vi "Functional Imaging-16bit display mapping.vi"(8 "error in (no error)":errorcluster) -> (0 "error out":errorcluster)   [LabVIEW 2013]
uses:
  Global variables/gl_Functional Imaging-Global variables.vi
panel:
  out "16-bit Display Mapping:All Elements":T1
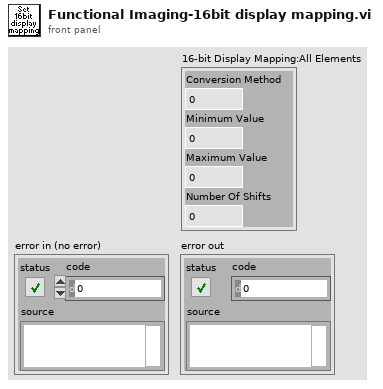
[diagram p1: front panel]
types:
  T1 = cluster{"Conversion Method":u32, "Minimum Value":i32, "Maximum Value":i32, "Number Of Shifts":i32}
  T2 = typedef "Functional Imging UI Refs.ctl" = cluster{"Menu ref":refnum<k9>, "Image control":refnum<vi>, "VI ref":refnum<vi>, "XGrapher":refnum<vi>, "Smoothing":refnum<vi>, "POI Averaging":refnum<vi>, "Normalize":refnum<vi>, "POI data points in each trial":refnum<vi>, "Channel":refnum<vi>, "Experiment data folder path":refnum<vi>, "[ROI vis]":refnum<vi>, "[Groups] visbl":T3, "Group Name":refnum<vi>, "POI index":refnum<vi>, "Trial No.":refnum<vi>, "Intensity Zoom":refnum<vi>, "Trial Cursor Enabled":refnum<vi>, "Number of Trials (ind 1)":refnum<vi>, "Number of Trials (ind 2)":refnum<vi>, "MiniScans Available":refnum<vi>, "POI Available":refnum<vi>, "Defer graph updates":refnum<vi>, "Waveform selector":refnum<vi>, "#of selected POI":refnum<vi>, "#of selected MiniScans":refnum<vi>, "#of selected groups":refnum<vi>, "Max Z-Projection":refnum<vi>, "Z-Plane Selector":refnum<vi>, "Index of miniscan point to visualise":refnum<vi>, "ROI vis. mode":refnum<vi>, "Total # of points":refnum<vi>, "Index of group clicked on":refnum<vi>, "Pane 1":refnum<vi>, "Pane 2":refnum<vi>, "Pane 3":refnum<vi>, "Pane 4":refnum<vi>, "Pane 5":refnum<vi>, "Pane 6":refnum<vi>, "Deselect all ROI":refnum<vi>, "Deselect all groups":refnum<vi>}
  T3 = typedef "Groups array referecne.ctl" = refnum<vi>
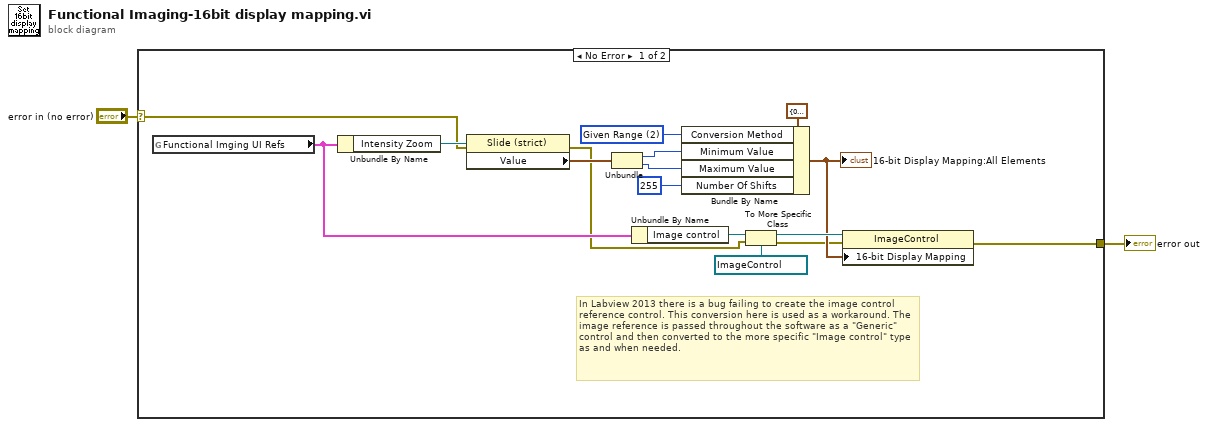
[diagram p0: block diagram]
diagram:
  n1 = case shown="No Error" "error in (no error)" {
    selector: "error in (no error)" -> [w3 w19]
    tunnel: [w4 w19] -> w2
    frame No Error {
      w16 = u32 2 items=["Full Dynamic", "Downshift", "Given Range", "90 % Dynamic", "Given Percent Range"] ("Conversion Method")
      # "In Labview 2013 there is a bug failing to create the image control reference control. This conversion here is used as a workaround. The image reference is passed throughout the software as a \"Generic\" control and then converted to the more specific \"Image control\" type as and when needed."
      n2 = global read "gl_Functional Imaging-Global variables.vi" "Functional Imging UI Refs"() -> (w9:T2)
      n3 = Unbundle By Name(w9) -> ("Intensity Zoom"=w17:refnum<vi>)
      n4 = property on="Property Node" class="Slide (strict)"(reference=w17, error in=w3) -> (error out=w6:errorcluster, "Value"=w18:cluster{u16, u16})  [unwired: 1 out]
      n5 = Unbundle(w18) -> (w15:u16, w14:u16)
      n6 = Unbundle By Name(w9) -> ("Image control"=w10:refnum<vi>)
      n7 = Bundle By Name(cluster=T1 {"Conversion Method"=0, "Minimum Value"=0, "Maximum Value"=0, "Number Of Shifts"=0} ("16-bit Display Mapping:All Elements"), "Conversion Method"=w16, "Minimum Value"=w15, "Maximum Value"=w14, "Number Of Shifts"=255) -> (w7:T1)
      "16-bit Display Mapping:All Elements" <- w7
      n8 = To More Specific Class(target class=refnum<vi> refnum ("Image"), reference=w10, error in=w6) -> (specific class reference=w8:refnum<vi>, error out=w5:errorcluster)
      n9 = property on="Property Node" class="ImageControl"(reference=w8, error in=w5, "16-bit Display Mapping"=w7) -> (error out=w4:errorcluster)  [unwired: 1 out]
    }
    frame Error {
    }
  }
  "error out" <- w2
